vi "Initialize From Settings.vi"(8 "error in (no error)":errorcluster, 9 "settings version":T1, 10 "settings":cluster{"key":string, "value":string}[](array[cluster]), 11 "UDP Rx Transfer Configuration in":refnum<class "UDP Transfer Rx Configuration.lvclass">) -> (0 "error out":errorcluster, 3 "UDP Rx Transfer Configuration out":refnum<class "UDP Transfer Rx Configuration.lvclass">)   [LabVIEW 2017, in "DSF Core.lvlib" / "UDP Transfer Rx Configuration.lvclass"]
uses:
  UDP Transfer Rx Configuration.lvclass
  Typedefs/DSF Version Info.ctl
  Rx Transfer Settings.ctl
  UDP Transfer Rx Configuration.lvclass/UDP Transfer Rx Configuration.ctl
  DSF Core.lvlib
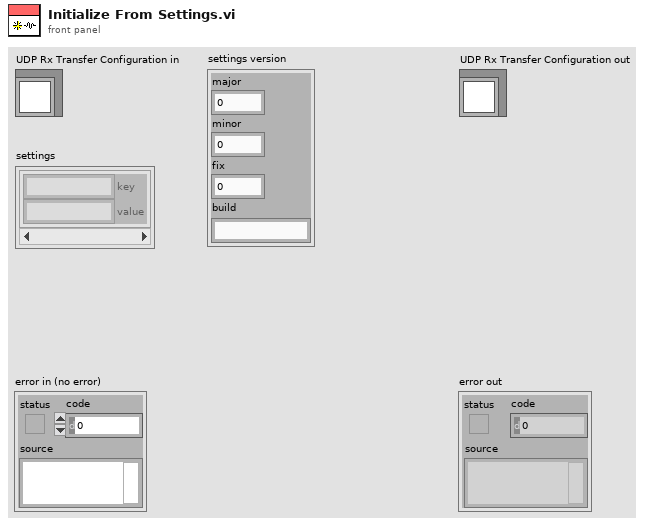
[diagram p1: front panel]
types:
  T1 = typedef "DSF Core.lvlib/DSF Version Info.ctl" = cluster{"major":u32, "minor":u32, "fix":u32, "build":string}
  T2 = typedef "DSF Core.lvlib/UDP Transfer Rx Configuration.lvclass/Rx Transfer Settings.ctl" = cluster{"address":u32, "port":u16}
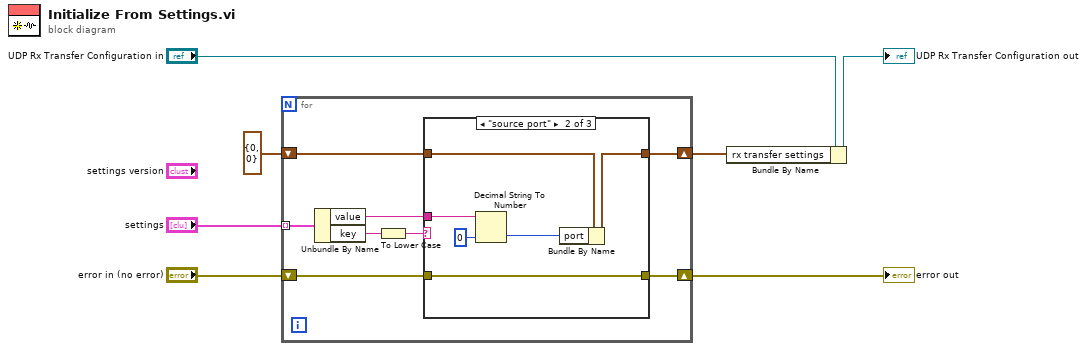
[diagram p0: block diagram]
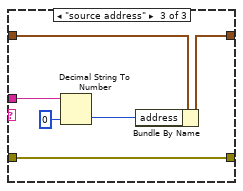
[diagram p3: hidden frame]
diagram:
  n1 = for {
    shift-right: [w8] -> w6
    shift-left: "error in (no error)" -> [w14]
    shift-right: [w10] -> w3
    shift-left: T2 {"address"=0, "port"=0} ("rx transfer settings") -> [w11]
    tunnel: "settings" -> [w15] mode=indexing
    n2 = Unbundle By Name(w15) -> ("value"=w12:string, "key"=w13:string)
    n3 = To Lower Case(string=w13) -> (all lower case string=w9:string)
    n4 = case shown="\"source port\"" w9 {
      tunnel: w14 -> [w16 w21 w27]
      tunnel: w12 -> [_ w20 w25]
      tunnel: w11 -> [w17 w23 w29]
      tunnel: [w17 w22 w28] -> w10
      tunnel: [w16 w21 w27] -> w8
      frame Default {
        # "Unknown Setting."
      }
      frame "source port" {
        n5 = Decimal String To Number(string=w20, default (0L)=u16 0 ("default (0 I32)")) -> (number=w19:u16)  [unwired: 1 in, 1 out]
        n6 = Bundle By Name(cluster=w23, "port"=w19) -> (w22:T2)
      }
      frame "source address" {
        n7 = Decimal String To Number(string=w25, default (0L)=u32 0 ("default (0 I32)")) -> (number=w24:u32)  [unwired: 1 in, 1 out]
        n8 = Bundle By Name(cluster=w29, "address"=w24) -> (w28:T2)
      }
    }
  }
  "error out" <- w6
  n9 = Bundle By Name(cluster="UDP Rx Transfer Configuration in", "rx transfer settings"=w3) -> (→"UDP Rx Transfer Configuration out":refnum<class "UDP Transfer Rx Configuration.lvclass">)
